vi "AutoScore-C.vi"(11 "Params":string[][](array[string])) -> ()   [LabVIEW 2019]
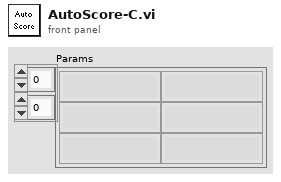
[diagram p1: front panel]
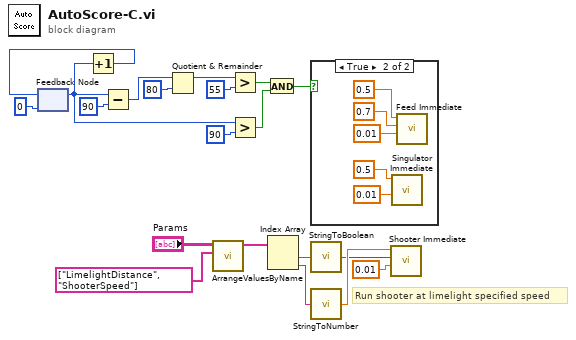
[diagram p0: block diagram]
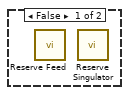
[diagram p2: hidden frame]
diagram:
  # "Run shooter at limelight specified speed"
  n1 = feedback #1(0) -> (w11:i32)
  n2 = Increment(x=w11) -> (x+1=w8:i32)
  n3 = feedback-in #1(w8) -> ()
  n4 = Subtract(x=w11, y=90) -> (x-y=w10:i32)
  n5 = Quotient & Remainder(x=w10, y=80) -> (x-y*floor(x/y)=w18:i32)  [unwired: 1 out]
  n6 = call "ArrangeValuesByName.vi"("Names"=string[] ["LimelightDistance", "ShooterSpeed"], "Names/Values in"="Params") -> ("Values Out"=w3:string[])  [unwired: 9 in]
  n7 = Greater?(x=w18, y=55) -> (0:w15:bool)
  n8 = Greater?(x=w11, y=90) -> (0:w14:bool)
  n9 = And(x=w15, y=w14) -> (x .and. y?=w9:bool)
  n10 = Index Array(array=w3) -> (element #1=w2:string, element #2=w1:string)  [unwired: 2 in]
  n11 = case shown="True" w9 {
    frame False {
      n12 = call "Reserve Feed.vi"() -> ()  [unwired: 11 in, 1 out]
      n13 = call "Reserve Singulator.vi"() -> ()  [unwired: 11 in, 1 out]
    }
    frame True {
      n14 = call "Singulator Immediate.vi"("Deadband"=0.01, "Setpoint"=0.5) -> ()  [unwired: 9 in, 1 out]
      n15 = call "Feed Immediate.vi"("Deadband Value"=0.01, "Upper Setpoint"=0.7, "Lower Setpoint"=0.5) -> ()  [unwired: 8 in, 1 out]
    }
  }
  n16 = call "StringToBoolean.vi"("String"=w2) -> ("Output"=w6:bool)
  n17 = call "StringToNumber.vi"("String"=w1) -> ("Output"=w7:dbl)
  n18 = call "Shooter Immediate.vi"("Deadband Value"=0.01, "LimeLightDistance?"=w6, "Setpoint"=w7) -> ()  [unwired: 8 in, 1 out]
